vi "Abort.vi"(8 "error in (no error)":errorcluster, 11 "MWWL Verification in":refnum<class "MWWL Verification.lvclass">) -> (0 "error out":errorcluster, 3 "MWWL Verification out":refnum<class "MWWL Verification.lvclass">)   [LabVIEW 2018, in "MWWL Verification.lvlib" / "MWWL Verification.lvclass"]
uses:
  MWWL Verification.lvclass
  MWWL Verification.lvclass/MWWL Verification.ctl
  <vilib>/ActorFramework/Message Enqueuer/Message Enqueuer.lvclass/Message Enqueuer.ctl
  <vilib>/ActorFramework/Message Enqueuer/Enqueue.vi
  <vilib>/ActorFramework/Stop Msg/Stop Msg.lvclass
  C:/Program Files (x86)/National Instruments/LabVIEW 2018/vi.lib/ActorFramework/Message/Message.lvclass
  <vilib>/ActorFramework/Message Priority Queue/Priority Enqueue.vi
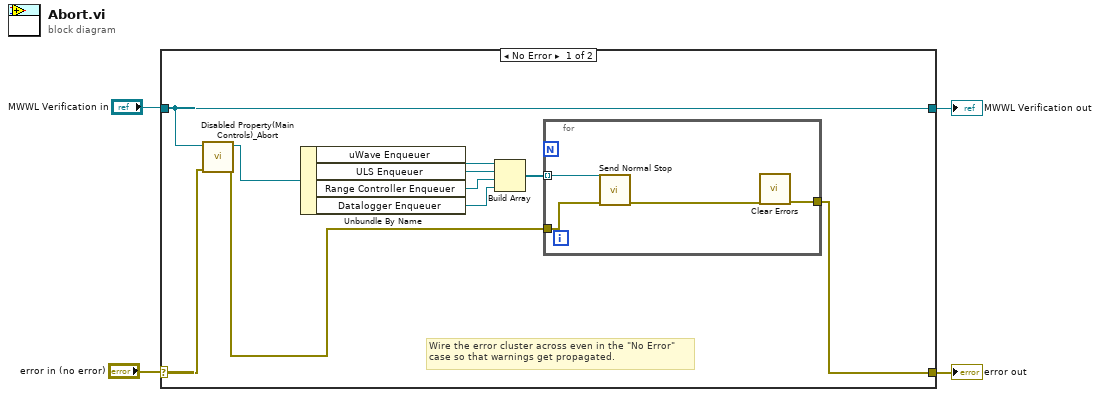
[diagram p0: block diagram]
diagram:
  n1 = case shown="No Error" "error in (no error)" {
    selector: "error in (no error)" -> [w7 w20]
    tunnel: [w14 w20] -> w3
    tunnel: [w9 w19] -> w1
    tunnel: "MWWL Verification in" -> [w9 w19]
    frame No Error {
      # "Wire the error cluster across even in the \"No Error\"\ncase so that warnings get propagated."
      n2 = call "Disabled Property(Main Controls)_Abort.vi"("error in (no error)"=w7, "MWWL Verification in"=w9) -> ("error out"=w6:errorcluster, "MWWL Verification out"=w8:refnum<class "MWWL Verification.lvclass">)  [unwired: 8 in]
      n3 = Unbundle By Name(w8) -> ("uWave Enqueuer"=w13:refnum<class "Message Enqueuer.lvclass">, "ULS Enqueuer"=w11:refnum<class "Message Enqueuer.lvclass">, "Range Controller Enqueuer"=w10:refnum<class "Message Enqueuer.lvclass">, "Datalogger Enqueuer"=w5:refnum<class "Message Enqueuer.lvclass">)
      n4 = Build Array(w13, w11, w10, w5) -> (w12:refnum<class "Message Enqueuer.lvclass">[])
      n5 = for {
        tunnel: [w18] -> w14
        tunnel: w12 -> [w17] mode=indexing
        tunnel: w6 -> [w16]
        n6 = call <vilib>:"Send Normal Stop.vi"("error in (no error)"=w16, "Message Enqueuer"=w17) -> ("error out"=w15:errorcluster)  [unwired: 9 in]
        n7 = call <vilib>:"Clear Errors.vi"("error in (no error)"=w15) -> ("error out"=w18:errorcluster)  [unwired: 5 in, 1 out]
      }
    }
    frame Error {
    }
  }
  "error out" <- w3
  "MWWL Verification out" <- w1
